vi "Uninit Menu.vi"(8 "error in (no error)":errorcluster, 11 "HamburgerMenu in":refnum<class "HamburgerMenu.lvclass">) -> (0 "error out":errorcluster, 3 "HamburgerMenu out":refnum<class "HamburgerMenu.lvclass">)   [LabVIEW 2017, in "Hamburger Menu Library.lvlib" / "HamburgerMenu.lvclass"]
uses:
  HamburgerMenu.lvclass
  HamburgerMenu.lvclass/HamburgerMenu.ctl
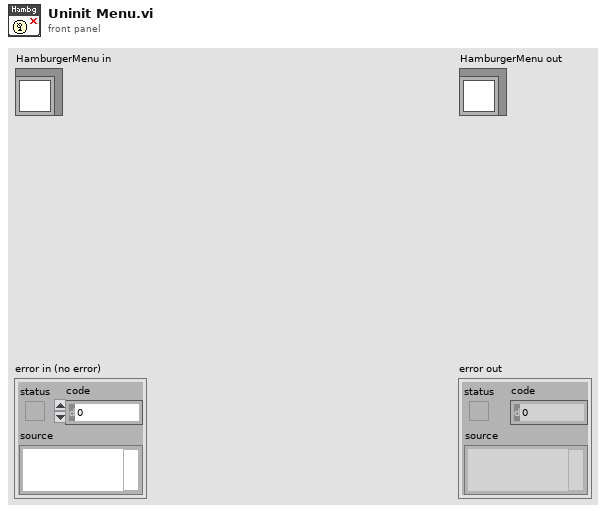
[diagram p1: front panel]
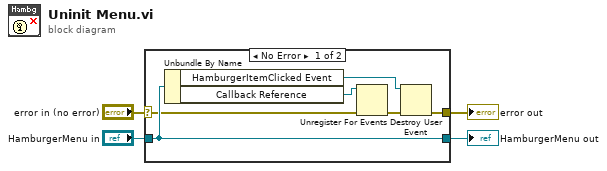
[diagram p0: block diagram]
diagram:
  n1 = case shown="No Error" "error in (no error)" {
    selector: "error in (no error)" -> [w6 w12]
    tunnel: [w5 w12] -> w3
    tunnel: [w10 w11] -> w1
    tunnel: "HamburgerMenu in" -> [w10 w11]
    frame No Error {
      n2 = Unbundle By Name(w10) -> ("HamburgerItemClicked Event"=w8:refnum<user-event>, "Callback Reference"=w9:refnum<k27>)
      n3 = Unregister For Events(event registration refnum=w9, error in=w6) -> (error out=w7:errorcluster)
      n4 = Destroy User Event(user event=w8, error in=w7) -> (error out=w5:errorcluster)
    }
    frame Error {
    }
  }
  "error out" <- w3
  "HamburgerMenu out" <- w1
